vi "Util_GetTime.vi"(8 "error in (no error)":i32, 11 "Pass_Through_Time":numeric format="%33.4f") -> (0 "error out":T1, 3 "FPGA_Time_Seconds":numeric format="%33.4f")   [LabVIEW 2019, in "Trajectory_Library.lvlib"]
doc: "This subVI returns the continuously running elapsed time in seconds. \n\nOn the RoboRIO this reads the high resolution FPGA time. The resolution, not accuracy, of the FPGA timer is 1 microsecond. The normal FPGA clock register (32 bits) rolls over approximately every 71 minutes. To significantly extend the rollover time,, this routine reads both the high and low FPGA clock registers. High/low register turnover read sequencing is dealt with by reading the high register twice, once before and once after the low register. If the values are different, the read is repeated to assure consistency between the high and low values. On a PC the standard operating system timer with 1 millisecond resolution is used. \n\nNotes:\n-------\n- On the RoboRIO this routine takes approximately 4.8 microseconds to execute. The WPI read FPGA clock routine takes approxmately 2.6 microseconds. The difference can be attributed to this routine reading to extra words from the FPGA. Each FPGA read takes approximately 1 microsecond. \n\n- Set a conditional complilation variable TRAJLIB_USEOSTIME and set it to a value of 1 to force this routine to read the RoboRIO operating system time instead of the FPGA time. This will have 1 millisecond resolution. This routine executes faster, approx 1 microsecond.\n\n - On the RoboRIO there is some drift between the FPGA and operating system clocks. The drift isn't consistent, but appears to be approximately 20 milliseconds / hour. This isn't enough to be of concern.\n\n\nParameters:\n - PassThroughTime -- If wired and the value is > 0 then this time is passed through and the FPGA time is not read. Allows calling functions to use a single time instant if desired.\n - Input Error -- Input error cluster\n\nReturns:\n - FPGA_Time_Seconds -- Elapsed time in seconds. \n - Output Error -- Output error cluster. An error will be returned if there are problems reading the FPGA or of the FPGA clock high register changes twice while reading the value.\n\nCustom Errors:\n - 8020 -- The upper FPGA time register changed during both attempts to read the FPGA time values. The returned time may not be valid."
uses:
  Trajectory_Library.lvlib
  <vilib>/Rock Robotics/SystemInterfaces/System/FPGA_SystemFRC FPGA Ref.ctl
  <vilib>/rvi/interface/nirviReadWriteControl/nirviReadWriteControl.xnode
  NiFpgaLv.dll
  <vilib>/Utility/error.llb/Error Cluster From Error Code.vi
  <vilib>/rvi/interface/Simulation/niFpgaSimulationCallBeginRW.vi
  <vilib>/rvi/errors/niLvFpgaAdjustHostInterfaceError.vi
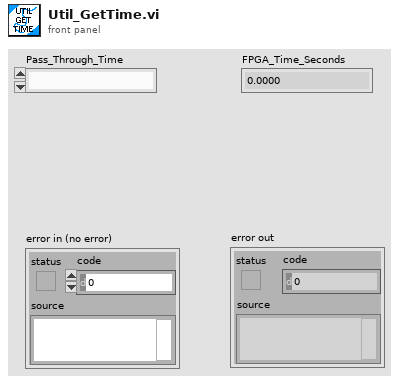
[diagram p1: front panel]
types:
  T1 = cluster{"source":string, "code":numeric, "status":boolean}
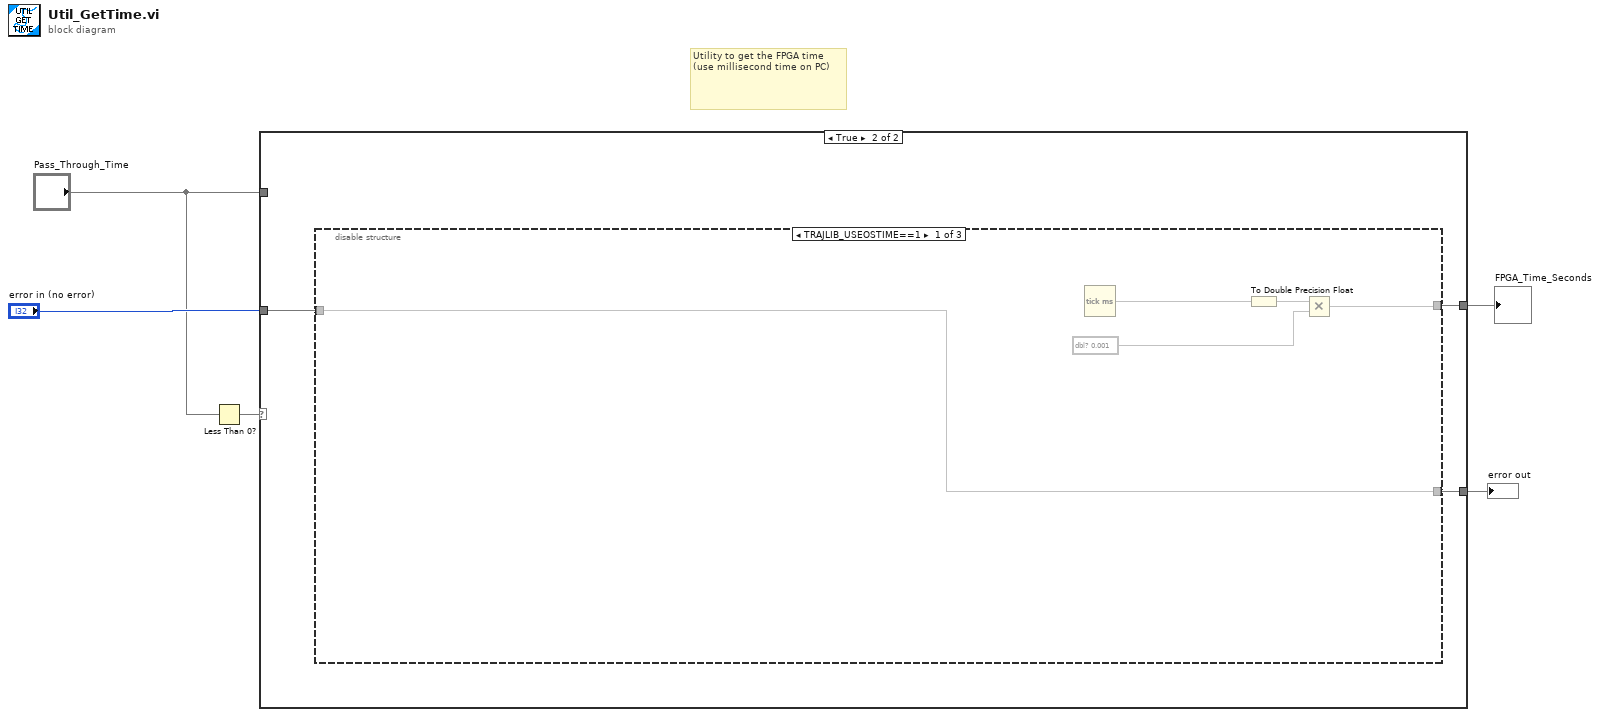
[diagram p0: block diagram]
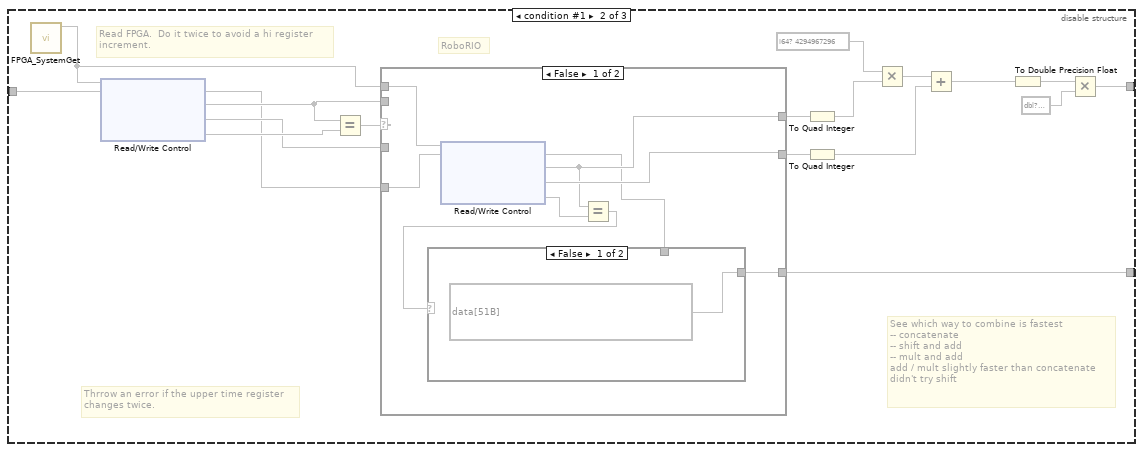
[diagram p3: hidden frame]
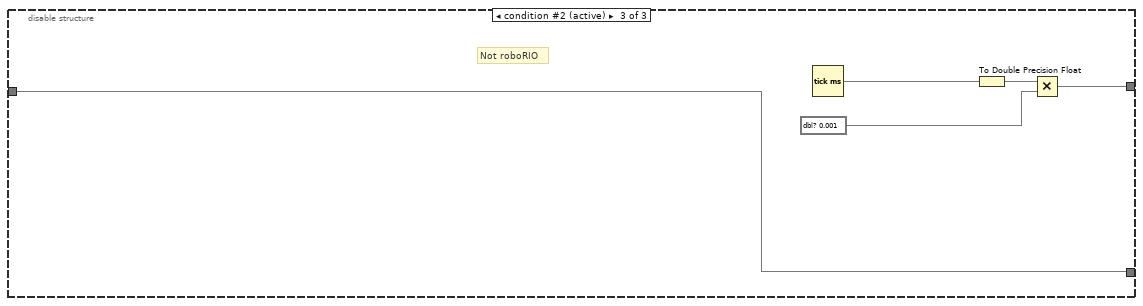
[diagram p6: hidden frame]
diagram:
  # "Utility to get the FPGA time\n(use millisecond time on PC)"
  n1 = Less Than 0?(x="Pass_Through_Time") -> (x < 0?=w2)
  n2 = case shown="True" w2 {
    tunnel: [w7 w10] -> w5
    tunnel: "error in (no error)" -> [w6 w9]
    tunnel: [w6 w8] -> w3
    tunnel: "Pass_Through_Time" -> [w7 _]
    frame 0 {
    }
    frame 1 {
      n3 = disable-structure shown="TRAJLIB_USEOSTIME==1" {
        disable-tunnel: [w12 w31 w48] -> w10
        disable-tunnel: w9 -> [w11 w16 w47]
        disable-tunnel: [w11 w19 w47] -> w8
        frame condition #0 {
          n4 = Tick Count (ms)() -> (millisecond timer value=w15)
          n5 = To Double Precision Float(number=w15) -> (double precision float=w14)
          n6 = Multiply(x=w14, y=dbl? 0.001) -> (x*y=w12)
        }
        frame condition #1 {
          # "See which way to combine is fastest\n-- concatenate\n-- shift and add\n-- mult and add\nadd / mult slightly faster than concatenate\ndidn't try shift"
          # "RoboRIO"
          # "Read FPGA.  Do it twice to avoid a hi register\nincrement."
          # "Thrrow an error if the upper time register\nchanges twice."
          n7 = call <vilib>:"FPGA_SystemGet.vi"() -> (3:w17)  [unwired: 11 in]
          n8 = xnode "Read/Write Control"(w17, w16) -> (w18, w22, w20, w30)  [unwired: 1 out]
          n9 = Equal?(x=w22, y=w30) -> (x = y?=w24)
          n10 = case shown="False" w24 {
            tunnel: [w38 w46] -> w23
            tunnel: w22 -> [_ w46]
            tunnel: [w39 w45] -> w21
            tunnel: w20 -> [_ w45]
            tunnel: [w35 w44] -> w19
            tunnel: w18 -> [w40 w44]
            tunnel: w17 -> [w41 _]
            frame 0 {
              n11 = xnode "Read/Write Control"(w41, w40) -> (w34, w38, w39, w37)  [unwired: 1 out]
              n12 = Equal?(x=w38, y=w37) -> (x = y?=w36)
              n13 = case shown="False" w36 {
                tunnel: [data[51B] ("error out") w43] -> w35
                tunnel: w34 -> [_ w43]
                frame 0 {
                }
                frame 1 {
                }
              }
            }
            frame 1 {
            }
          }
          n14 = To Quad Integer(1:w23) -> (0:w26)
          n15 = To Quad Integer(1:w21) -> (0:w25)
          n16 = Multiply(x=i64? 4294967296, y=w26) -> (x*y=w29)
          n17 = Add(x=w29, y=w25) -> (x+y=w27)
          n18 = To Double Precision Float(number=w27) -> (double precision float=w32)
          n19 = Multiply(x=w32, y=dbl? 1e-06) -> (x*y=w31)
        }
        frame condition #2 (active) {
          # "Not roboRIO"
          n20 = Tick Count (ms)() -> (millisecond timer value=w51)
          n21 = To Double Precision Float(number=w51) -> (double precision float=w50)
          n22 = Multiply(x=w50, y=dbl? 0.001) -> (x*y=w48)
        }
      }
    }
  }
  "FPGA_Time_Seconds" <- w5
  "error out" <- w3
